vi "TDVM Analyze Time Domain Measurements.vi"(0 "Voltage Waveforms In":waveform(dbl)[](array[waveform]), 5 "Periodic Waveform \nMeasurements":bool=TRUE, 11 "error in (no error)":errorcluster) -> (4 "Time Domain Measurements":T1 {"Voltage Waveform duty cycle (%)" format="%#.2p"; "Voltage Waveform Period (s)" format="%#.2p"; "Voltage Frequency(Hz)" format="%#.2p"; "Vpp Amplitude(V)" format="%#.2p"; "Mean DC Voltage (V)" format="%#.2p"}, 15 "error out":errorcluster)   [LabVIEW 2021, in "DAQ_Time Domain Measurement.lvlib"]
doc: "Analyzes the voltage waveforms data obtained from analog input voltage measurements to derive required time domain measurements"
uses:
  DAQ_Time Domain Measurement.lvlib
  Typedefs/Time Domain Measurements.ctl
  <vilib>/measure/mascope.llb/Amplitude and Levels N chan.vi
  <vilib>/measure/madcrms.llb/Basic Averaged DC-RMS for N Chan.vi
  <vilib>/measure/mascope.llb/Pulse Measurements N chan.vi
  <vilib>/measure/NI_MAPro.lvlib
panel:
  # "Inputs"
  # "Outputs"
  # "Overview:\nThis VI does post processing on obtained voltage waveforms from analog input voltage measurements to give the required time domain Measurements output\n\nInstructions:\n1. Input the captured voltage waveforms to the input controls\n2. Observe the analyzed time domain measurements output"
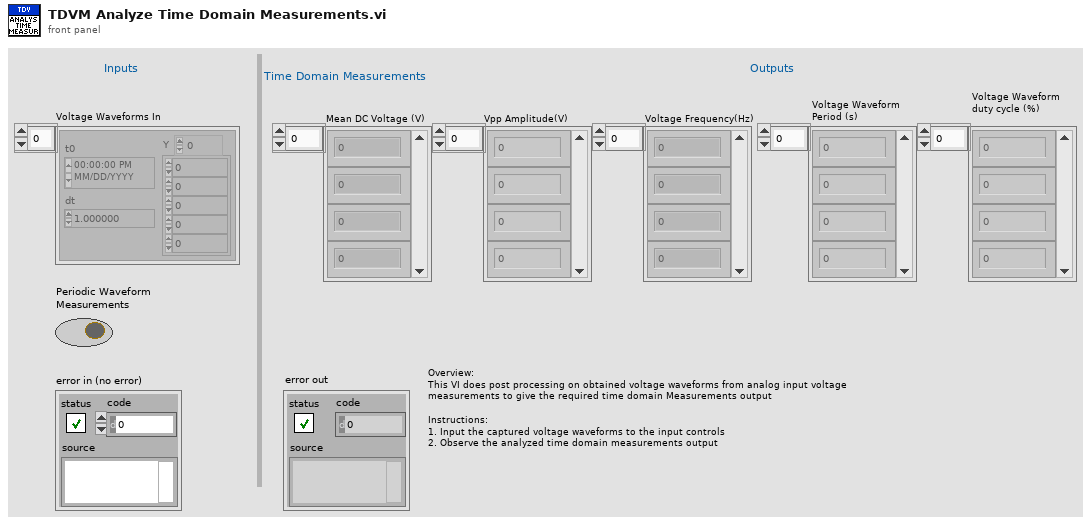
[diagram p1: front panel]
types:
  T1 = typedef "DAQ_Time Domain Measurement.lvlib/Time Domain Measurements.ctl" = cluster{"Mean DC Voltage (V)":dbl[], "Vpp Amplitude(V)":dbl[], "Voltage Frequency(Hz)":dbl[], "Voltage Waveform Period (s)":dbl[], "Voltage Waveform duty cycle (%)":dbl[]}
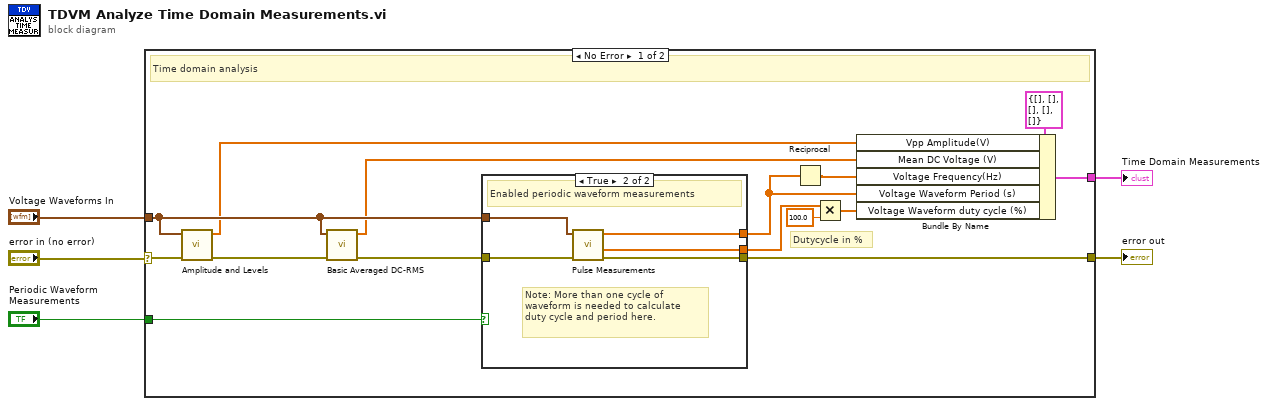
[diagram p0: block diagram]
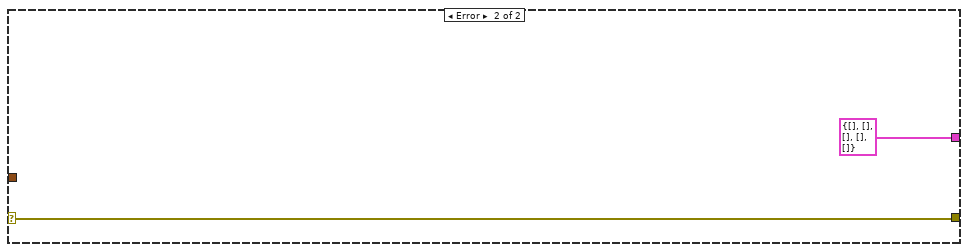
[diagram p3: hidden frame]
diagram:
  n1 = case shown="No Error" "error in (no error)" {
    selector: "error in (no error)" -> [w14 w28]
    tunnel: "Voltage Waveforms In" -> [w19 _]
    tunnel: [w17 T1 {"Mean DC Voltage (V)"=[], "Vpp Amplitude(V)"=[], "Voltage Frequency(Hz)"=[], "Voltage Waveform Period (s)"=[], "Voltage Waveform duty cycle (%)"=[]} ("Measure Settings")] -> w3
    tunnel: [w16 w28] -> w2
    tunnel: "Periodic Waveform \nMeasurements" -> [w11 _]
    frame No Error {
      # "Dutycycle in %"
      # "Time domain analysis"
      n2 = call-poly <vilib>:"Amplitude and Levels.vi"("error in (no error)"=w14, "signal(s) in"=w19) -> ("error out"=w20:errorcluster, "amplitude"=w10:dbl[])  [unwired: 6 in, 2 out]
      n3 = call-poly <vilib>:"Basic Averaged DC-RMS.vi"("error in (no error)"=w20, "signals in"=w19) -> ("error out"=w15:errorcluster, "DC values"=w9:dbl[])  [unwired: 6 in, 2 out]
      n4 = case shown="True" w11 {
        tunnel: w19 -> [_ w26]
        tunnel: [_ w25] -> w7
        tunnel: [w21 w24] -> w16
        tunnel: w15 -> [w21 w23]
        tunnel: [_ w22] -> w13
        frame False {
          # "Disabled periodic waveform measurements"
        }
        frame True {
          # "Note: More than one cycle of waveform is needed to calculate\nduty cycle and period here."
          # "Enabled periodic waveform measurements"
          n5 = call-poly <vilib>:"Pulse Measurements.vi"("error in (no error)"=w23, "signal(s) in"=w26) -> ("error out"=w24:errorcluster, "duty cycle"=w25:dbl[], "period"=w22:dbl[])  [unwired: 5 in, 2 out]
        }
      }
      n6 = Reciprocal(x=w13) -> (1/x=w12:dbl[])
      n7 = Multiply(x=w7, y=100.0) -> (x*y=w8:dbl[])
      n8 = Bundle By Name(cluster=T1 {"Mean DC Voltage (V)"=[], "Vpp Amplitude(V)"=[], "Voltage Frequency(Hz)"=[], "Voltage Waveform Period (s)"=[], "Voltage Waveform duty cycle (%)"=[]} ("Measure Settings"), "Vpp Amplitude(V)"=w10, "Mean DC Voltage (V)"=w9, "Voltage Frequency(Hz)"=w12, "Voltage Waveform Period (s)"=w13, "Voltage Waveform duty cycle (%)"=w8) -> (w17:T1)
    }
    frame Error {
    }
  }
  "error out" <- w2
  "Time Domain Measurements" <- w3
